vi "Complete Request.vi"(7 "Processing In":refnum<class "Processing.lvclass">, 11 "WebSocket Handler in":refnum<class "WebSocket Handler.lvclass">) -> (0 "error out":errorcluster, 5 "Processing":refnum<class "Processing.lvclass">)   [LabVIEW 2020, in "HTTP Server.lvlib" / "WebSocket Handler.lvclass"]
uses:
  WebSocket Handler.lvclass
  Processing/Processing.lvclass
  Processing/Processing.lvclass/Processing.ctl
  lv-stream-websocket/Stream-Websocket/Websocket Server/Websocket Server.lvclass
  C:/dev/lv20CE/relink/lv-stream/stream/Endpoint/Endpoint.lvclass
  WebSocket Handler.lvclass/WebSocket Handler.ctl
  lv-http-util/HTTP Utils/Request/Request.lvclass
  lv-stream/stream/Endpoint/Endpoint.lvclass
  lv-uri/URI/URI/URI.lvclass
  lv-stream/stream/URI/URI.lvclass
  C:/dev/lv20CE/relink/lv-stream-websocket/Stream-Websocket/Websocket Server/Websocket Server.lvclass
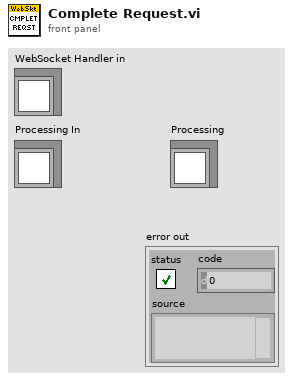
[diagram p1: front panel]
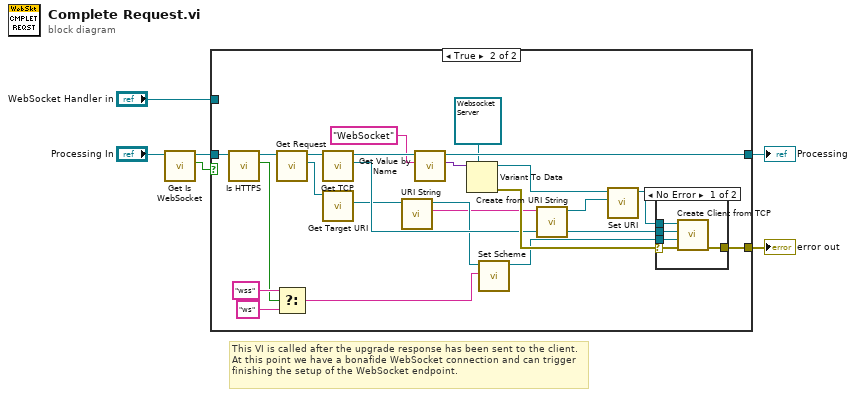
[diagram p0: block diagram]
diagram:
  # "This VI is called after the upgrade response has been sent to the client. At this point we have a bonafide WebSocket connection and can trigger finishing the setup of the WebSocket endpoint."
  n1 = call "Get Is WebSocket.vi"("Processing in"="Processing In") -> ("Is WebSocket"=w6:bool, "Processing out"=w5:refnum<class "Processing.lvclass">)  [unwired: 9 in]
  n2 = case shown="True" w6 {
    tunnel: w5 -> [w7 w28]
    tunnel: [w7 w19] -> w3
    tunnel: "WebSocket Handler in" -> [_ _]
    tunnel: [_ w22] -> w1
    frame False {
    }
    frame True {
      n3 = call "Is HTTPS.vi"("Processing in"=w28) -> ("HTTPS?"=w25:bool, "Processing out"=w21:refnum<class "Processing.lvclass">)  [unwired: 8 in, 1 out]
      n4 = call "Get Request.vi"("Processing in"=w21) -> ("Request"=w18:refnum<class "Request.lvclass">, "Processing out"=w20:refnum<class "Processing.lvclass">)  [unwired: 9 in]
      n5 = Select(t="wss", s=w25, f="ws") -> (s? t:f=w24:string)
      n6 = call "Get TCP.vi"("Processing in"=w20) -> ("TCP"=w12:refnum<k5>, "Processing out"=w29:refnum<class "Processing.lvclass">)  [unwired: 9 in]
      n7 = call "Get Target URI.vi"("Request in"=w18) -> ("Target URI"=w11:refnum<class "URI.lvclass">)  [unwired: 8 in, 2 out]
      n8 = call "URI String.vi"("URI in"=w11) -> ("URI String"=w9:string, "URI"=w10:refnum<class "URI.lvclass">)  [unwired: 9 in]
      n9 = call "Get Value by Name.vi"("Name"="WebSocket" ("Name for Type"), "Processing in"=w29) -> ("Value"=w16:variant, "Processing out"=w19:refnum<class "Processing.lvclass">)  [unwired: 7 in, 1 out]
      n10 = Variant To Data(type=refnum<class "Websocket Server.lvclass"> refnum ("WebSocket"), Variant=w16) -> (data=w14:refnum<class "Websocket Server.lvclass">, error out=w30:errorcluster)  [unwired: 1 in]
      n11 = call "Set Scheme.vi"("Scheme"=w24, "URI in"=w10) -> ("URI out"=w23:refnum<class "URI.lvclass">)  [unwired: 9 in]
      n12 = call "Create from URI String.vi"("URI String"=w9) -> ("URI out"=w8:refnum<class "URI.lvclass">)  [unwired: 9 in, 1 out]
      n13 = call "Set URI.vi"("URI"=w8, "Endpoint in"=w14) -> ("Endpoint out"=w17:refnum<class "Websocket Server.lvclass">)  [unwired: 8 in, 1 out]
      n14 = case shown="No Error" w30 {
        selector: w30 -> [w32 w36]
        tunnel: w17 -> [w35 _]
        tunnel: w12 -> [w34 _]
        tunnel: w23 -> [w33 _]
        tunnel: [w31 w36] -> w22
        frame No Error {
          n15 = call "Create Client from TCP.vi"("error in (no error)"=w32, "URI"=w33, "TCP Connection"=w34, "Websocket Server in"=w35) -> ("error out"=w31:errorcluster)  [unwired: 6 in, 1 out]
        }
        frame Error {
        }
      }
    }
  }
  "error out" <- w1
  "Processing" <- w3
